vi "Stock_MP.vi"() -> ()   [LabVIEW 2024]
panel:
  in  "Stock MP":dbl
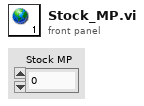
[diagram p1: front panel]
diagram:
